vi "Create a new bucket.vi"() -> ()   [LabVIEW 2011]
doc: "This example demonstrates the use of the Create bucket API call.\n\n<B>!!! NOTE : For some reason, currently you cannot use the default US Classic region. !!!\nIf you want to use this operation, read through the whole Create VI Documentation, because the above restriction causes other guidelines you have to follow!</B>\n\nTo use this example, <B>you must register with Amazon S3 and have a valid AWS Access Key ID</B> to authenticate requests."
uses:
  vi.lib/National Instruments/LabVIEW Interface for Amazon S3/Typedefs/AMZ_S3_LocationConstraint.ctl
  Typedefs/Access_Key_Type.ctl
  Typedefs/Secret_Key_Type.ctl
  vi.lib/National Instruments/LabVIEW Interface for Amazon S3/Typedefs/AMZ_S3_AWS Credentials.ctl
  vi.lib/National Instruments/LabVIEW Interface for Amazon S3/Typedefs/AMZ_S3_API_PUT Bucket Request Parameters.ctl
  vi.lib/National Instruments/LabVIEW Interface for Amazon S3/Typedefs/AMZ_S3_ACL.ctl
  vi.lib/National Instruments/LabVIEW Interface for Amazon S3/LV Interface for Amazon S3.lvlib
panel:
  in  "Secret Key":T1
  in  "Access Key":T2
  in  "stop":bool
  in  "Create":bool
  in  "Random":bool
  in  "Bucket name":string
  in  "Location":T3=enum."US-West-1"
  # "To use this VI, you have to register first with Amazon to have an Amazon AWS account.\nIf you don't have an account yet, go to http://aws.amazon.com and Create an AWS account!"
  # "If you want to make a bucket in Amazon's default, US Classic region, you have to create it using another method!\nGo to \"https://console.aws.amazon.com/s3/home\" to access the AWS Console, where you can create the bucket."
  # "1. Fill in your AWS Credentials\n2. Run this VI\n3. You can modify the Location to create the bucket in another Region\n4. Fill in a Bucket name, or Press Random name button any number of times to generate random names\n\n!!! The bucket name has to be globally unique !!!\n\n5. Press Create button to Create the bucket"
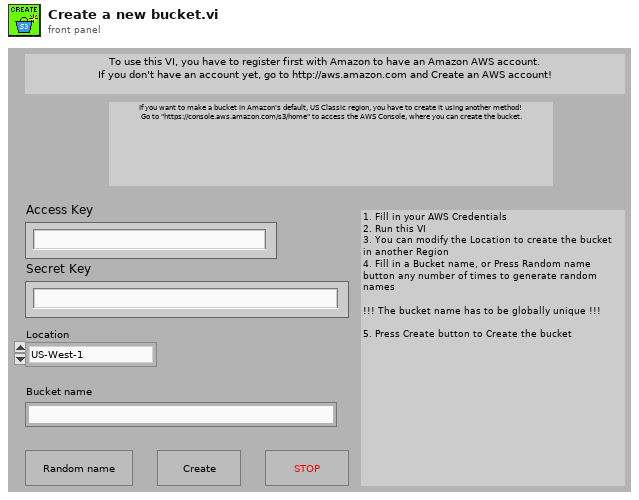
[diagram p1: front panel]
types:
  T1 = typedef "Secret_Key_Type.ctl" = string
  T2 = typedef "Access_Key_Type.ctl" = string
  T3 = typedef "LV Interface for Amazon S3.lvlib/AMZ_S3_LocationConstraint.ctl" = enum16{"US Classic", "EU", "US-West-1", "AP-SouthEast-1"}
  T4 = typedef "LV Interface for Amazon S3.lvlib/AMZ_S3_AWS Credentials.ctl" = cluster{"Access Key":string, "Secret Key":string}
  T5 = typedef "LV Interface for Amazon S3.lvlib/AMZ_S3_API_PUT Bucket Request Parameters.ctl" = cluster{"ACL":T6, "Location":T3}
  T6 = typedef "LV Interface for Amazon S3.lvlib/AMZ_S3_ACL.ctl" = enum16{"private", "public-read", "public-read-write", "authenticated-read", "bucket-owner-read", "bucket-owner-full-control"}
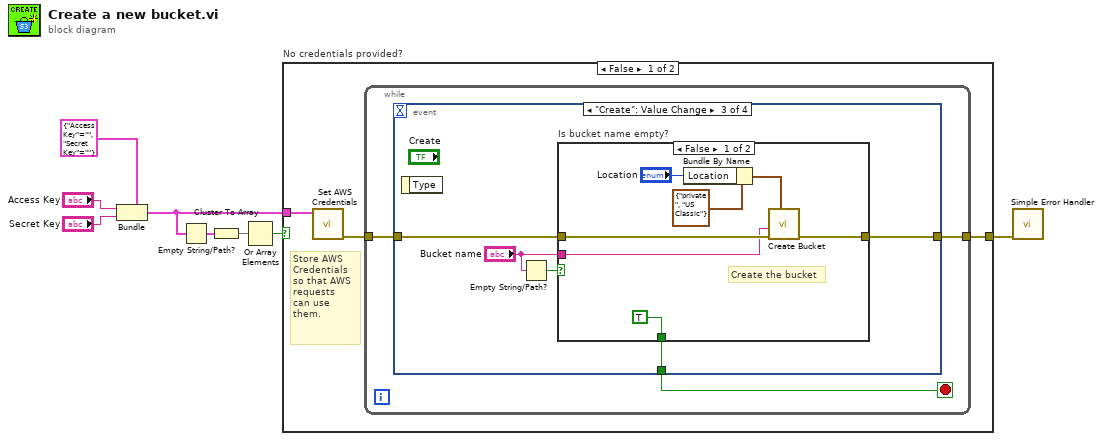
[diagram p0: block diagram]
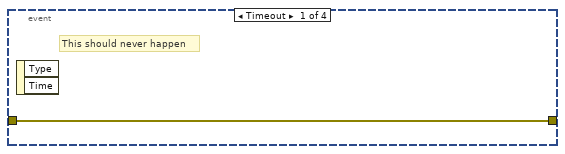
[diagram p2: hidden frame]
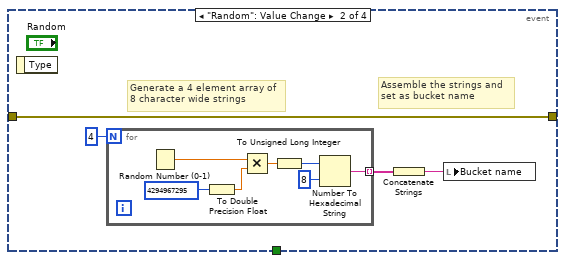
[diagram p3: hidden frame]
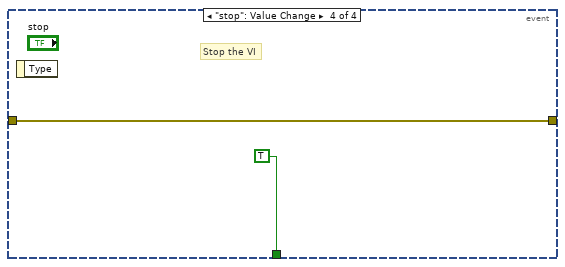
[diagram p5: hidden frame]
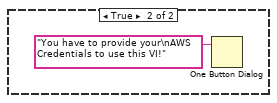
[diagram p6: hidden frame]
diagram:
  n1 = Bundle(cluster=T4 {"Access Key"="", "Secret Key"=""} ("AWS Credentials in"), "Access Key"="Access Key", "Secret Key"="Secret Key") -> (w1:T4)
  n2 = Empty String/Path?(string/path=w1) -> (empty?=w8:cluster{"Access Key":bool, "Secret Key":bool})
  n3 = Cluster To Array(cluster=w8) -> (array=w7:bool[])
  n4 = Or Array Elements(Boolean array=w7) -> (logical OR=w6:bool)
  n5 = case "No credentials provided?" shown="False" w6 {
    tunnel: w1 -> [w11 _]
    tunnel: [w9 _] -> w5
    frame False {
      # "Store AWS Credentials\nso that AWS requests\ncan use them."
      n6 = call "Set AWS Credentials.vi"("AWS Credentials in"=w11) -> ("error out"=w10:errorcluster)  [unwired: 10 in]
      n7 = while {
        tunnel: w10 -> [w14]
        tunnel: [w12] -> w9
        stop <- w13 stop-if-true
        n8 = event shown="[2] \"Create\": Value Change" {
          selector: _ -> [_ _ _ _]
          dyn-events: _ -> [_ _ _ _]
          timeout: _ -> [_ _ _ _]
          tunnel: w14 -> [w15 w17 w31 w40]
          tunnel: [_ _ w27 TRUE] -> w13
          tunnel: [w15 w17 w28 w40] -> w12
          event Timeout {
            # "This should never happen"
            n9 = event-data() -> ()  [unwired: 1 in, 2 out]
          }
          event "Random": Value Change {
            # "Assemble the strings and\nset as bucket name"
            # "Generate a 4 element array of\n8 character wide strings"
            n10 = event-data() -> ()  [unwired: 1 in, 1 out]
            n11 = for {
              N: 4 -> [_]
              tunnel: [w20] -> w18 mode=indexing
              n12 = Random Number (0-1)() -> (number: 0 to 1=w26:dbl)
              n13 = To Double Precision Float(number=u32 4294967295) -> (double precision float=w24:dbl)
              n14 = Multiply(x=w26, y=w24) -> (x*y=w23:dbl)
              n15 = To Unsigned Long Integer(number=w23) -> (unsigned 32bit integer=w22:u32)
              n16 = Number To Hexadecimal String(1:i16 8 ("width (-)"), 2:w22) -> (0:w20:string)
            }
            n17 = Concatenate Strings(w18) -> (w16:string)
            n18 = local write "Bucket name"(w16) -> ()
          }
          event "Create": Value Change {
            n19 = event-data() -> ()  [unwired: 1 in, 1 out]
            n20 = Empty String/Path?(string/path="Bucket name") -> (empty?=w30:bool)
            n21 = case "Is bucket name empty?" shown="False" w30 {
              tunnel: w31 -> [w36 w39]
              tunnel: "Bucket name" -> [w35 _]
              tunnel: [w33 w39] -> w28
              tunnel: [TRUE _] -> w27
              frame False {
                # "Create the bucket"
                n22 = Bundle By Name(cluster=T5 {"ACL"=enum."private", "Location"=enum."US Classic"} ("Request parameters"), "Location"="Location") -> (w34:T5)
                n23 = call "Create Bucket.vi"("Request parameters"=w34, "error in (no error)"=w36, "Bucket"=w35) -> ("error out"=w33:errorcluster)  [unwired: 8 in]
              }
              frame True {
                # "Do nothing"
              }
            }
          }
          event "stop": Value Change {
            # "Stop the VI"
            n24 = event-data() -> ()  [unwired: 1 in, 1 out]
          }
        }
      }
    }
    frame True {
      n25 = One Button Dialog(message="You have to provide your\nAWS Credentials to use this VI!") -> ()  [unwired: 1 in, 1 out]
    }
  }
  n26 = call <vilib>:"Simple Error Handler.vi"("error in (no error)"=w5) -> ()  [unwired: 4 in, 5 out]
